vi "Measure.vi"(6 "Init work":bool, 7 "Update period":dbl, 8 "error in (no error)":errorcluster, 9 "Last request":bool, 10 "Requester":string, 11 "Continuous Recorder Actor in":refnum<class "Continuous Recorder Actor.lvclass">) -> (0 "error out":errorcluster, 3 "Continuous Recorder Actor out":refnum<class "Continuous Recorder Actor.lvclass">)   [LabVIEW 2021, in "Continuous Recorder Actor.lvclass"]
uses:
  Continuous Recorder Actor.lvclass
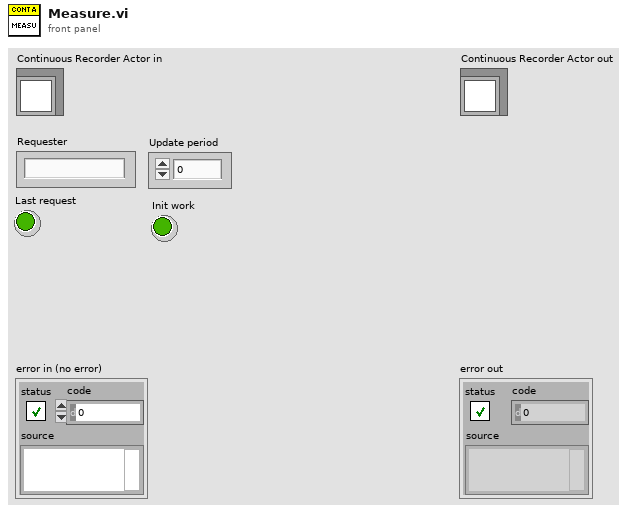
[diagram p1: front panel]
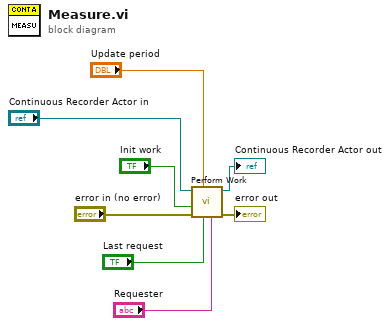
[diagram p0: block diagram]
diagram:
  n1 = call-dynamic "Perform Work.vi"("Controller name"="Requester", "Last request"="Last request", "Update period"="Update period", "error in (no error)"="error in (no error)", "Initialize"="Init work", "Measure Object in"="Continuous Recorder Actor in") -> ("error out"=→"error out":errorcluster, "Measure Object out"=→"Continuous Recorder Actor out":refnum<class "Continuous Recorder Actor.lvclass">)  [unwired: 4 in]
